vi "Plot Names Tester.vi"() -> ()   [LabVIEW 2010]
doc: "이 VI는 플롯 이름 설정 VI를 테스트하는데 사용됩니다."
panel:
  in  "플롯 이름":string[](array[string])
  out "웨이브폼 그래프":dbl[](graph)
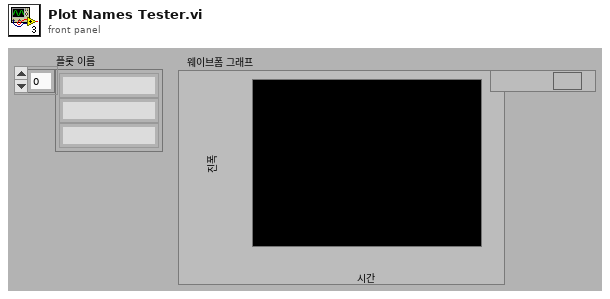
[diagram p1: front panel]
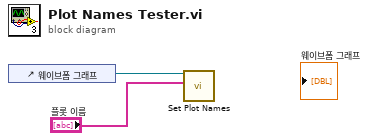
[diagram p0: block diagram]
diagram:
  n1 = control-ref of="웨이브폼 그래프"() -> (w1:refnum<vi>)
  n2 = call "Set Plot Names.vi"("플롯 이름"="플롯 이름", "그래프 참조"=w1) -> ()  [unwired: 9 in, 1 out]
